vi "TimeOut Timer 2.vi"(8 "error in (no error)":errorcluster, 9 "Message":T1, 11 "Timer":refnum<queue>) -> (0 "error out":errorcluster)   [LabVIEW 2014]
uses:
  Engine/Message.ctl
  support/Message Queue/Message Cluster.ctl
  Teszt/Teszt.ctl
  Teszt/Command.ctl
  support/Message Queue/Enqueue Message (Single).vi
  support/Message Queue/Message Queue.lvlib
panel:
  out "Elipsed Timer (ms)":u32
  out "Time has Elapsed":bool
  out "Numeric Control":i32
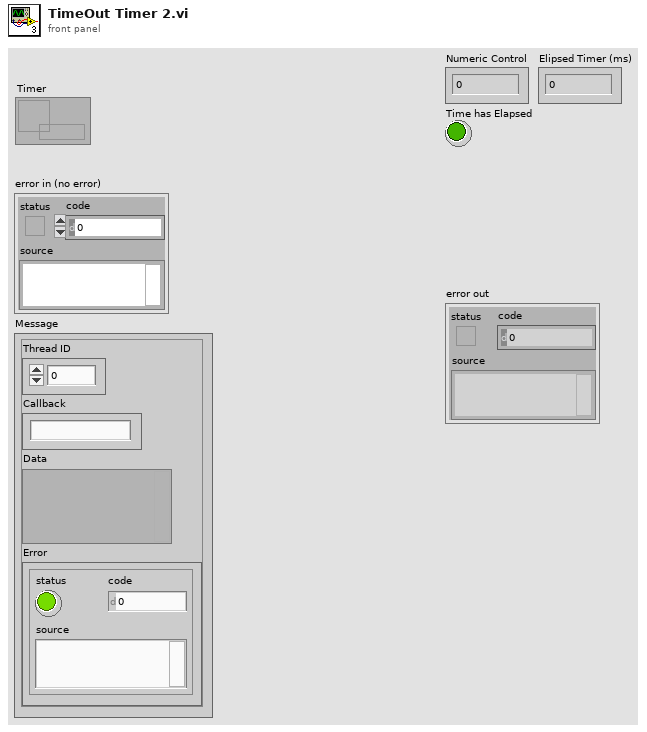
[diagram p1: front panel]
types:
  T1 = typedef "Message.ctl" = cluster{"Thread ID":u16, "Callback":string, "Data":variant, "Error":errorcluster}
  T2 = typedef "Teszt.ctl" = cluster{"Thread ID":dbl, "Mérésszám":string, "Mérés/Utasítás":string, "Command":T3, "Min":string, "Max":string, "Aktív?":bool, "Log?":bool, "Kiértékelés":bool, "Etalon 1 exp":bool, "Etalon 2 exp":bool, "Etalon 3 exp":bool, "Etalon 4 exp":bool, "Etalon 5 exp":bool}
  T3 = typedef "Command.ctl" = cluster{"Parancs":string, "Paraméter 1":string, "Paraméter 2":string, "Paraméter 3":string, "Paraméter 4":string, "Paraméter 5":string, "Eredmény":string}
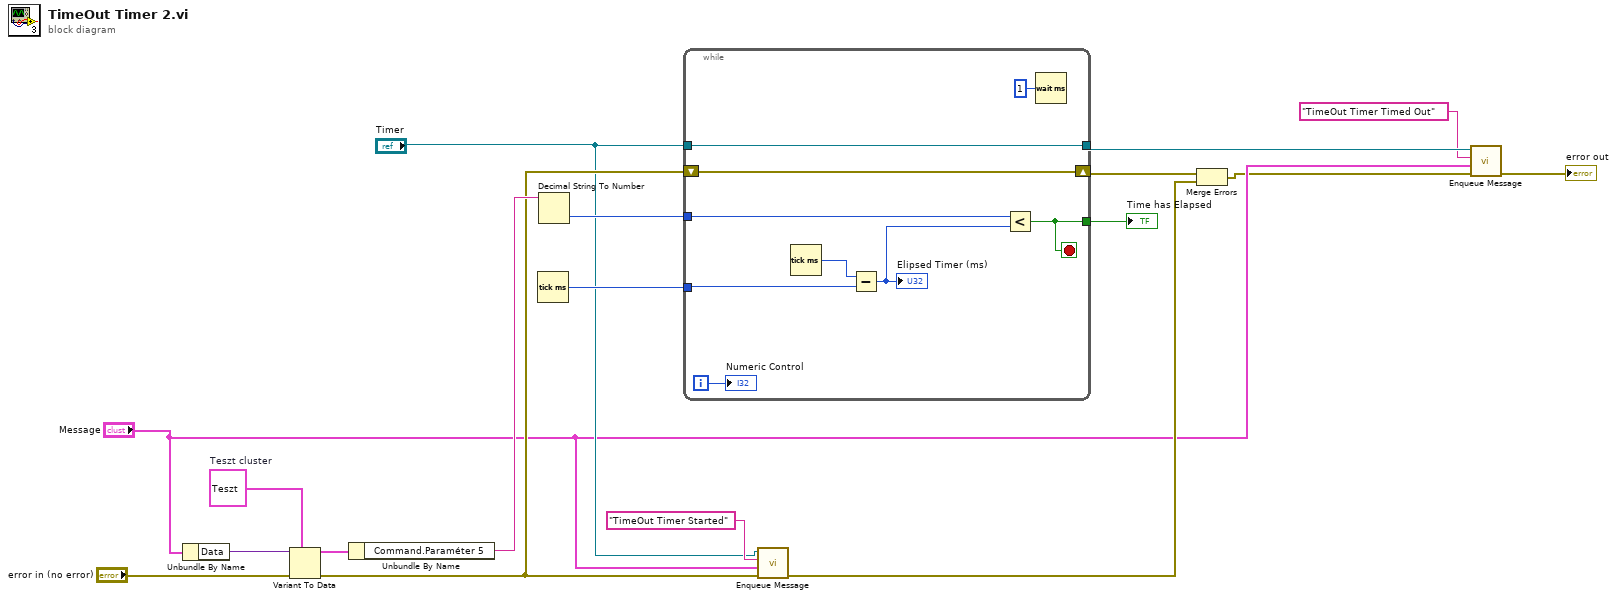
[diagram p0: block diagram]
diagram:
  w15 = T2 {"Thread ID"=0.0, "Mérésszám"="", "Mérés/Utasítás"="", "Command"={"Parancs"="", "Paraméter 1"="", "Paraméter 2"="", "Paraméter 3"="", "Paraméter 4"="", "Paraméter 5"="", "Eredmény"=""}, "Min"="", "Max"="", "Aktív?"=FALSE, "Log?"=FALSE, "Kiértékelés"=FALSE, "Etalon 1 exp"=FALSE, "Etalon 2 exp"=FALSE, "Etalon 3 exp"=FALSE, "Etalon 4 exp"=FALSE, "Etalon 5 exp"=FALSE}  # Teszt cluster
  n1 = Unbundle By Name("Message") -> ("Data"=w14:variant)
  n2 = Variant To Data(error in="error in (no error)", type=w15, Variant=w14) -> (data=w13:T2, error out=w6:errorcluster)
  n3 = Unbundle By Name(w13) -> ("Command.Paraméter 5"=w12:string)
  n4 = Tick Count (ms)() -> (millisecond timer value=w10:u32)
  n5 = Decimal String To Number(string=w12) -> (number=w9:i32)  [unwired: 2 in, 1 out]
  n6 = while {
    tunnel: [w27] -> w18
    tunnel: "Timer" -> [w27]
    shift-right: [w19] -> w4
    shift-left: w6 -> [w19]
    tunnel: w10 -> [w23]
    tunnel: w9 -> [w22]
    tunnel: [w20] -> w8
    i -> [w25]
    stop <- w20 stop-if-true
    n7 = Tick Count (ms)() -> (millisecond timer value=w24:u32)
    n8 = Subtract(x=w24, y=w23) -> (x-y=w21:u32)
    "Elipsed Timer (ms)" <- w21
    n9 = Less?(x=w22, y=w21) -> (x < y?=w20:bool)
    n10 = Wait (ms)(milliseconds to wait=u32 1) -> ()  [unwired: 1 out]
    "Numeric Control" <- w25
  }
  "Time has Elapsed" <- w8
  n11 = call-poly "Enqueue Message.vi"("error in (no error)"=w6, "Message Data"="Message", "Message"="TimeOut Timer Started", "Message Queue"="Timer") -> ("error out"=w3:errorcluster)  [unwired: 6 in, 1 out]
  n12 = Merge Errors(w4, w3) -> (w1:errorcluster)
  n13 = call-poly "Enqueue Message.vi"("error in (no error)"=w1, "Message Data"="Message", "Message"="TimeOut Timer Timed Out", "Message Queue"=w18) -> ("error out"=→"error out":errorcluster)  [unwired: 6 in, 1 out]
